vi "Quadrature.vi"() -> ()   [LabVIEW 2013]
uses:
  <vilib>/Rock Robotics/SystemInterfaces/Typedef/FPGA_TypedefDigitalModule.ctl
  <vilib>/Rock Robotics/SystemInterfaces/DIO/FPGA_DIOChannel.ctl
  <vilib>/Rock Robotics/WPI/Encoder/WPI_EncoderType.ctl
  <vilib>/Rock Robotics/WPI/Counter/WPI_CounterDigitalInputToDigitalSource.vi
panel:
  out "Distance":dbl
  out "B":bool
  out "A":bool
  out "Stopped":bool
  out "Speed":dbl(graph)
  out "Distance":dbl(graph)
  out "Direction":bool
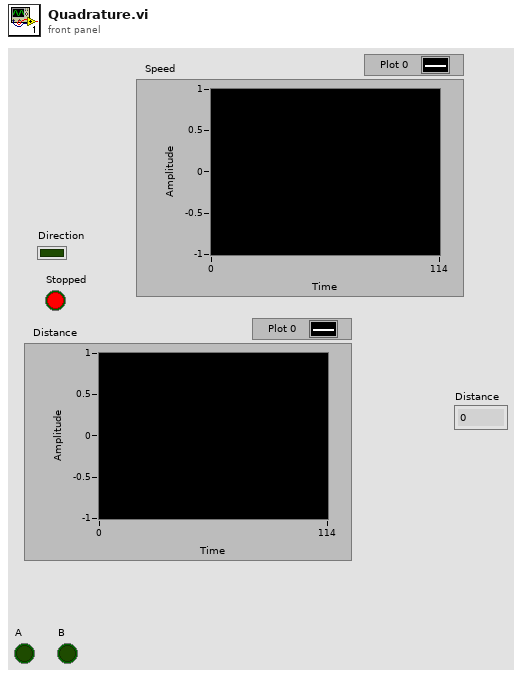
[diagram p1: front panel]
types:
  T1 = typedef "WPI_EncoderType.ctl" = enum16{"1x", "2x", "4x"}
  T2 = typedef "FPGA_DIOChannel.ctl" = enum8{"DIO 1", "DIO 2", "DIO 3", "DIO 4", "DIO 5", "DIO 6", "DIO 7", "DIO 8", "DIO 9", "DIO 10", "DIO 11", "DIO 12", "DIO 13", "DIO 14", "Invalid"}
  T3 = typedef "FPGA_TypedefDigitalModule.ctl" = enum16{"Digital Module 1", "Digital Module 2"}
  T4 = typedef "WPI_DigitalInputDevRef.ctl" = cluster{"DevStatus":errorcluster, "DIO Channel":T2, "Digital Module":T3}
  T5 = typedef "FPGA_CounterEncoderSourceConvertionLVSourceType.ctl" = cluster{"DevStatus":errorcluster, "AnalogTriggerMode?":bool, "DigitalMode":cluster{"Digital Module":T3, "DIO Channel":T6}, "AnalogTriggerMode":cluster{"AnalogTriggerIndex":T7, "OutputType":T8}}
  T6 = typedef "FPGA_DIODigitalSourceChannel.ctl" = enum8{"DIO 1", "DIO 2", "DIO 3", "DIO 4", "DIO 5", "DIO 6", "DIO 7", "DIO 8", "DIO 9", "DIO 10", "DIO 11", "DIO 12", "DIO 13", "DIO 14", "Disabled"}
  T7 = typedef "FPGA_AnalogTriggerIndex.ctl" = enum8{"Trig 0", "Trig 1", "Trig 2", "Trig 3", "Trig 4", "Trig 5", "Trig 6", "Trig 7", "Invalid"}
  T8 = typedef "FPGA_AnalogTriggerOutType.ctl" = enum16{"InWindow", "TriggerState", "Rising", "Falling"}
  T9 = typedef "WPI_EncoderDevRef.ctl" = cluster{"DevStatus":errorcluster, "EncoderIndex":T10, "CounterIndex":T11, "DistancePerCount":dbl, "Decoding Type":T1}
  T10 = typedef "FPGA_EncoderIdx.ctl" = enum8{"Enc 0", "Enc 1", "Enc 2", "Enc 3", "Invalid"}
  T11 = typedef "FPGA_CounterCtrSystemIndex.ctl" = enum8{"Ctr 0", "Ctr 1", "Ctr 2", "Ctr 3", "Ctr 4", "Ctr 5", "Ctr 6", "Ctr 7", "Invalid"}
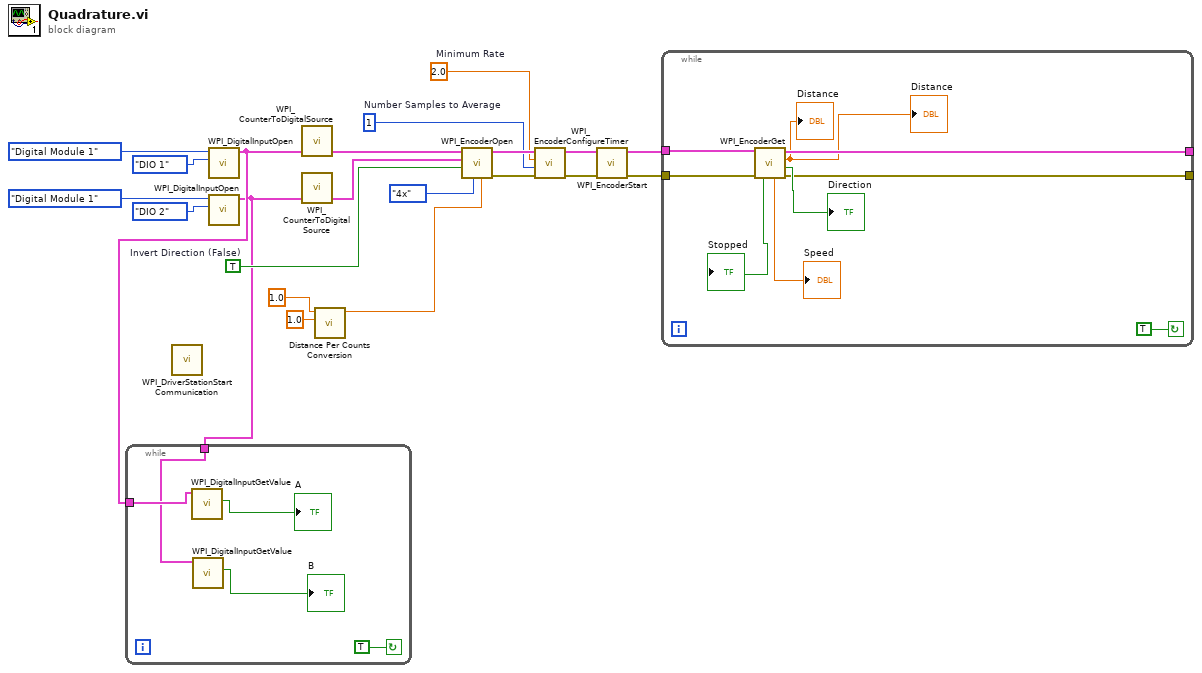
[diagram p0: block diagram]
diagram:
  w11 = TRUE  # Invert Direction (False)
  w13 = u8 1  # Number Samples to Average
  w14 = 2.0  # Minimum Rate
  n1 = call <vilib>:"WPI_DriverStationStart Communication.vi"() -> ()  [unwired: 12 in]
  n2 = call <vilib>:"WPI_DigitalInputOpen.vi"("DIO Channel"=FPGA_DIOChannel."DIO 1", "Digital Module (Module 1)"=FPGA_TypedefDigitalModule."Digital Module 1") -> ("DigitalInputDevRef"=w6:T4)  [unwired: 1 in, 8 out]
  n3 = call <vilib>:"WPI_DigitalInputOpen.vi"("DIO Channel"=FPGA_DIOChannel."DIO 2", "Digital Module (Module 1)"=FPGA_TypedefDigitalModule."Digital Module 1") -> ("DigitalInputDevRef"=w5:T4)  [unwired: 1 in, 8 out]
  n4 = while {
    tunnel: w6 -> [w24]
    tunnel: w5 -> [w23]
    stop <- TRUE continue-if-true
    n5 = call <vilib>:"WPI_DigitalInputGetValue.vi"("DigitalInputDevRef"=w24) -> ("Value"=→"A":bool)  [unwired: 8 in, 2 out]
    n6 = call <vilib>:"WPI_DigitalInputGetValue.vi"("DigitalInputDevRef"=w23) -> ("Value"=→"B":bool)  [unwired: 8 in, 2 out]
  }
  n7 = call-poly <vilib>:"WPI_CounterToDigitalSource.vi"("DigitalInputDevRef"=w6) -> ("Digital Source"=w20:T5)  [unwired: 6 out]
  n8 = call-poly <vilib>:"WPI_CounterToDigitalSource.vi"("DigitalInputDevRef"=w5) -> ("Digital Source"=w21:T5)  [unwired: 6 out]
  n9 = call "Distance Per Counts Conversion.vi"("Counts Per Rev"=1.0, "WheelDiameter"=1.0) -> ("Distance/Count"=w9:dbl)  [unwired: 9 in]
  n10 = call <vilib>:"WPI_EncoderOpen.vi"("DistancePerCount"=w9, "Decoding Type"=WPI_EncoderType."4x", "Invert Direction (False)"=w11, "BSource"=w21, "ASource"=w20) -> ("error out"=w10:errorcluster, "EncoderDevRef"=w17:T9)  [unwired: 3 in, 2 out]
  n11 = call <vilib>:"WPI_EncoderConfigureTimer.vi"("error in (no error)"=w10, "Number Samples to Average"=w13, "Minimum Rate"=w14, "EncoderDevRef"=w17) -> ("error out"=w4:errorcluster, "EncoderDevRef"=w3:T9)  [unwired: 6 out]
  n12 = call <vilib>:"WPI_EncoderStart.vi"("error in (no error)"=w4, "EncoderDevRef"=w3) -> ("error out"=w1:errorcluster, "EncoderDevRef"=w2:T9)  [unwired: 8 in]
  n13 = while {
    tunnel: w2 -> [w33]
    tunnel: w1 -> [w34]
    tunnel: [w32] -> _
    tunnel: [w30] -> _
    stop <- TRUE continue-if-true
    n14 = call <vilib>:"WPI_EncoderGet.vi"("error in (no error)"=w34, "EncoderDevRef"=w33) -> ("error out"=w30:errorcluster, "Direction"=→"Direction":bool, "Distance"=→"Distance" →"Distance":dbl, "EncoderDevRef"=w32:T9, "Rate"=→"Speed":dbl, "Stopped"=→"Stopped":bool)  [unwired: 4 in]
  }
